vi "6.3_FileReader.vi"() -> ()   [LabVIEW 2025]
panel:
  out "String Read from Path":string
  in  "File Path":path
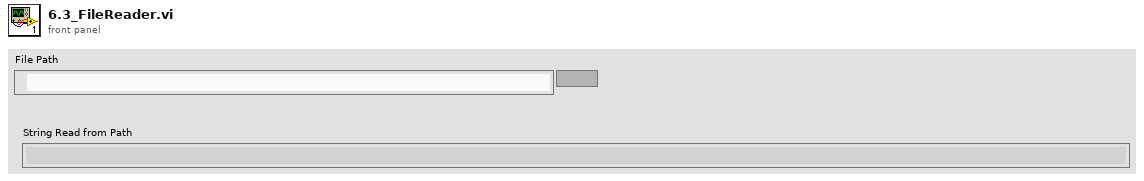
[diagram p1: front panel]
types:
  T1 = enum16{"open", "replace", "create", "open or create", "replace or create", "replace or create with confirmation"}
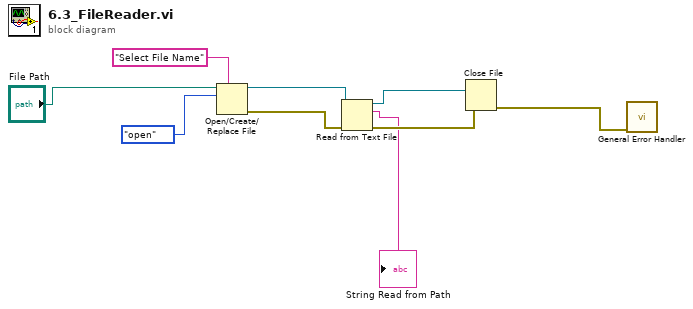
[diagram p0: block diagram]
diagram:
  n1 = Open/Create/Replace File(file path (use dialog)="File Path", prompt="Select File Name", operation (0:open)=T1."open") -> (refnum out=w2:refnum<file>, error out=w9:errorcluster)  [unwired: 3 in, 1 out]
  n2 = Read from Text File(file (use dialog)=w2, error in=w9) -> (refnum out=w1:refnum<file>, text=→"String Read from Path":string, error out=w8:errorcluster)  [unwired: 2 in, 1 out]
  n3 = Close File(refnum=w1, error in=w8) -> (error out=w7:errorcluster)  [unwired: 1 out]
  n4 = call <vilib>:"General Error Handler.vi"("error in (no error)"=w7) -> ()  [unwired: 10 in, 5 out]
